vi "Initialize Attribute Channels.vi"(8 "error in (no error)":errorcluster, 10 "Number of Channels":i32, 11 "CS++FgenChannelData in":refnum<class "CS++FgenChannelData.lvclass">) -> (0 "error out":errorcluster, 3 "CS++FgenChannelData out":refnum<class "CS++FgenChannelData.lvclass">)   [LabVIEW 2015, in "CS++FgenGui.lvlib" / "CS++FgenChannelData.lvclass"]
doc: "Initalize Attribute array with default number of channels."
uses:
  CS++FgenChannelData.lvclass
  CS++FgenChannelData.lvclass/CS++FgenChannelData.ctl
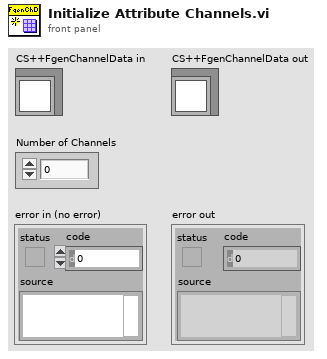
[diagram p1: front panel]
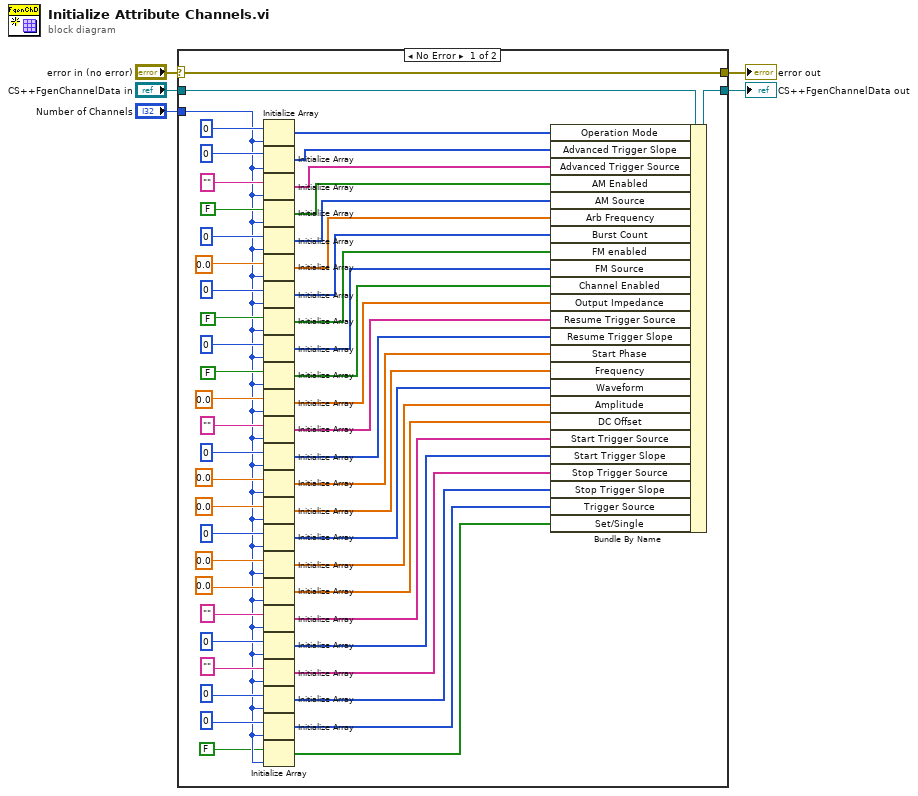
[diagram p0: block diagram]
diagram:
  n1 = case shown="No Error" "error in (no error)" {
    selector: "error in (no error)" -> [w57 w59]
    tunnel: [w57 w59] -> w4
    tunnel: [w55 w58] -> w2
    tunnel: "CS++FgenChannelData in" -> [w56 w58]
    tunnel: "Number of Channels" -> [w8 _]
    frame No Error {
      n2 = Initialize Array(0 ("operation mode (Continuous)"), w8) -> (w53:i32[])
      n3 = Initialize Array(0 ("Trigger Slope (Positive)"), w8) -> (w51:i32[])
      n4 = Initialize Array("" ("Trigger Source (None)"), w8) -> (w49:string[])
      n5 = Initialize Array(FALSE ("AM enabled (True)"), w8) -> (w47:bool[])
      n6 = Initialize Array(0 ("source (Internal)"), w8) -> (w45:i32[])
      n7 = Initialize Array(dbl[unit] 0.0 ("frequency (0.0 Hz)"), w8) -> (w43:dbl[unit][])
      n8 = Initialize Array(0 ("burst count (1)"), w8) -> (w41:i32[])
      n9 = Initialize Array(FALSE ("FM enabled (True)"), w8) -> (w39:bool[])
      n10 = Initialize Array(0 ("source (Internal)"), w8) -> (w37:i32[])
      n11 = Initialize Array(FALSE ("channel enabled (True)"), w8) -> (w35:bool[])
      n12 = Initialize Array(dbl[unit] 0.0 ("impedance (50 Ohms)"), w8) -> (w33:dbl[unit][])
      n13 = Initialize Array("" ("Trigger Source (None)"), w8) -> (w31:string[])
      n14 = Initialize Array(0 ("Trigger Slope (Positive)"), w8) -> (w29:i32[])
      n15 = Initialize Array(dbl[unit] 0.0 ("start phase (0.00 Degrees)"), w8) -> (w27:dbl[unit][])
      n16 = Initialize Array(dbl[unit] 0.0 ("frequency (1000.0 Hz)"), w8) -> (w25:dbl[unit][])
      n17 = Initialize Array(0 ("waveform (Sine)"), w8) -> (w23:i32[])
      n18 = Initialize Array(dbl[unit] 0.0 ("amplitude (1.00 V)"), w8) -> (w21:dbl[unit][])
      n19 = Initialize Array(dbl[unit] 0.0 ("dc offset (0.00 V)"), w8) -> (w19:dbl[unit][])
      n20 = Initialize Array("" ("Trigger Source (None)"), w8) -> (w17:string[])
      n21 = Initialize Array(0 ("Trigger Slope (Positive)"), w8) -> (w15:i32[])
      n22 = Initialize Array("" ("Trigger Source (None)"), w8) -> (w13:string[])
      n23 = Initialize Array(0 ("Trigger Slope (Positive)"), w8) -> (w11:i32[])
      n24 = Initialize Array(0 ("trigger source (External)"), w8) -> (w9:i32[])
      n25 = Initialize Array(FALSE ("channel enabled (True)"), w8) -> (w6:bool[])
      n26 = Bundle By Name(cluster=w56, "Operation Mode"=w53, "Advanced Trigger Slope"=w51, "Advanced Trigger Source"=w49, "AM Enabled"=w47, "AM Source"=w45, "Arb Frequency"=w43, "Burst Count"=w41, "FM enabled"=w39, "FM Source"=w37, "Channel Enabled"=w35, "Output Impedance"=w33, "Resume Trigger Source"=w31, "Resume Trigger Slope"=w29, "Start Phase"=w27, "Frequency"=w25, "Waveform"=w23, "Amplitude"=w21, "DC Offset"=w19, "Start Trigger Source"=w17, "Start Trigger Slope"=w15, "Stop Trigger Source"=w13, "Stop Trigger Slope"=w11, "Trigger Source"=w9, "Set/Single"=w6) -> (w55:refnum<class "CS++FgenChannelData.lvclass">)
    }
    frame Error {
    }
  }
  "error out" <- w4
  "CS++FgenChannelData out" <- w2
